vi "fft_test.vi"() -> ()   [LabVIEW 2016]
uses:
  xcontrol/Start Button.xctl
  <vilib>/silver_ctls/ArrayMatrixCluster/Real Matrix NI_Silver.ctl
  <vilib>/Instr/_visa.llb/VISA Configure Serial Port (Instr).vi
  <instrlib>/Tektronix TDS 200 1000 2000 Series/Public/Data/Read (Single Waveform).vi
  <instrlib>/Tektronix TDS 200 1000 2000 Series/Tektronix TDS 200 1000 2000 Series.lvlib
panel:
  out "OSC ERR":bool=TRUE
  in  "Vertical Range (10.0 V/div)":dbl=0.005 format="%^1_3g"
  out "Waveform Graph":dbl[](graph)
  in  "Sampling Frequency":dbl=500000.0
  in  "Number of Sample":i32=2500
  out "Ölçülen Sinyal":dynamicdata(graph)
  out "Real Matrix":T1
  out "İlk Ayar":bool=TRUE
  out "Osc Data":waveform(dbl)(graph)
  in  "Osiloskop Portu":refnum<visa-resource-name>="USB0::0x0699::0x0363::C102985::INSTR"
  in  "Start Button":dbl(xcontrol)
  in  "Frekans (kHz)":i32(slide)=100 caption="Amplitude(V)" step=1 scale=0.0..100.0
  in  "Reset Dafault":bool
  in  "Teta":i32(slide) scale=0.0..360.0
  in  "Sinyal Jeneratörü Portu":refnum<visa-resource-name>="COM4"
  in  "OUTPUT":bool=TRUE caption="Output"
  in  "Offset":i32(slide) scale=0.0..10.0
  in  "Amplitude(V)":i32(slide)=20 scale=0.0..20.0
  in  "cmdOrjin":bool
  in  "cmdStop":bool
  # "R-O Tarayıcı ile Bilgisayar Kontrollü Halka Anten Radyasyon Paterni Ölçüm Düzeneği Geliştirilmesi"
  # "Frekans"
  # "Teta"
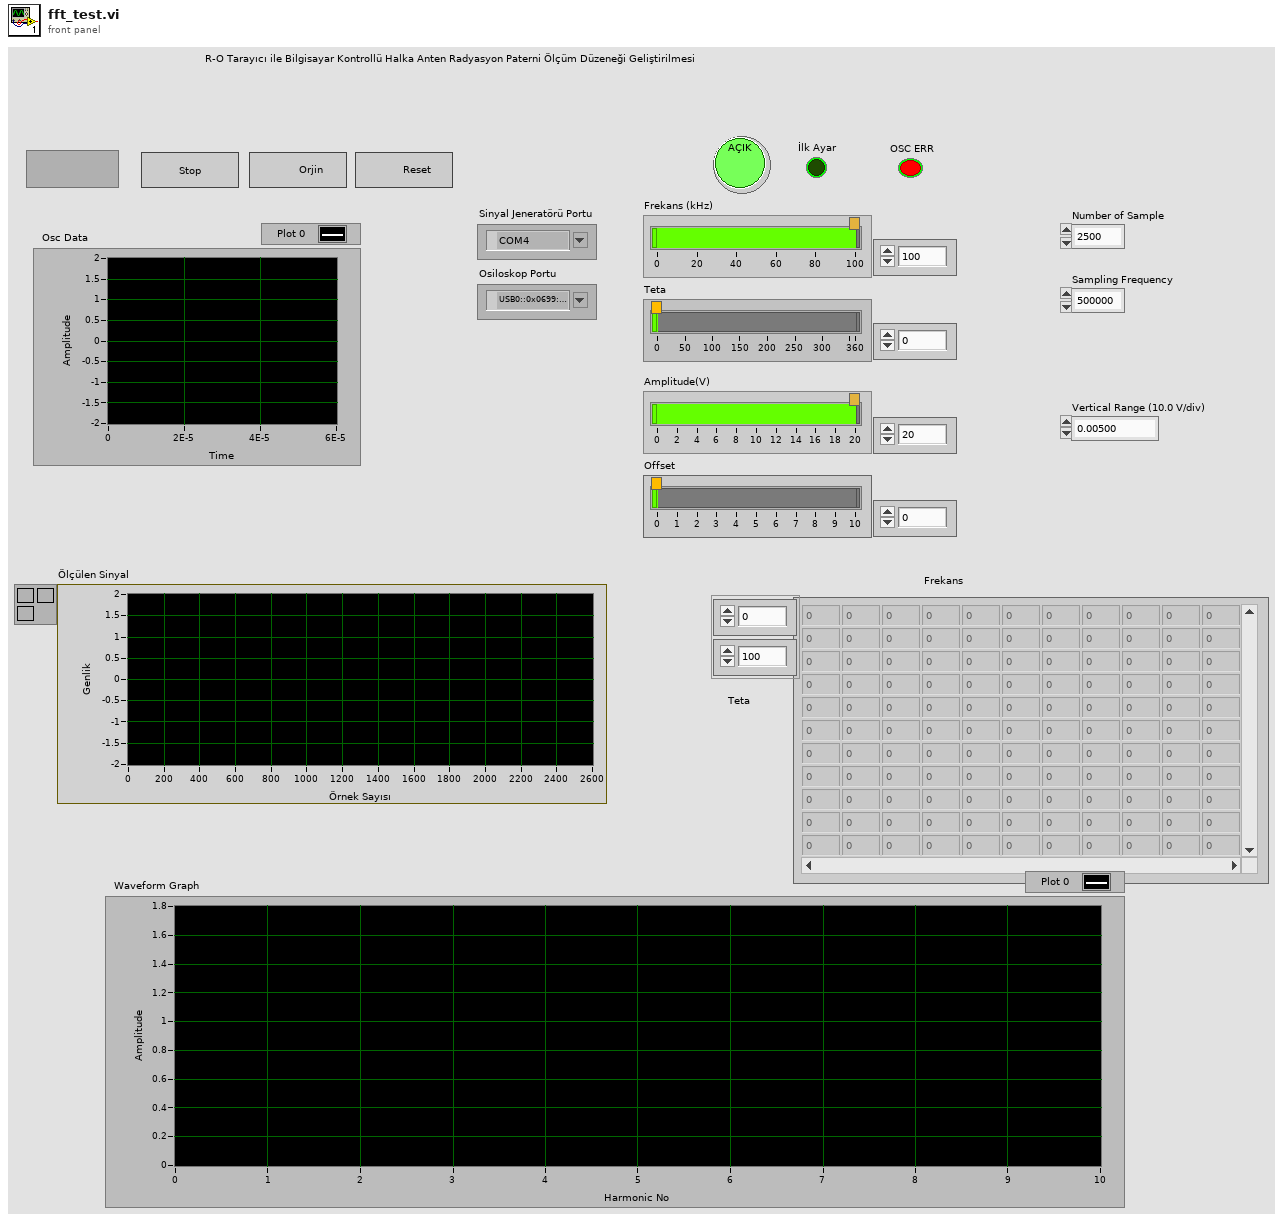
[diagram p1: front panel]
types:
  T1 = typedef "Real Matrix NI_Silver.ctl" = dbl[][]
  T2 = cluster{"Baud Rate":u32, "Parity":u16, "Stop Bits":u16, "Flow Control":u16}
  T3 = typedef "NI_Matrix.lvlib/RealMatrix.ctl" = dbl[][]
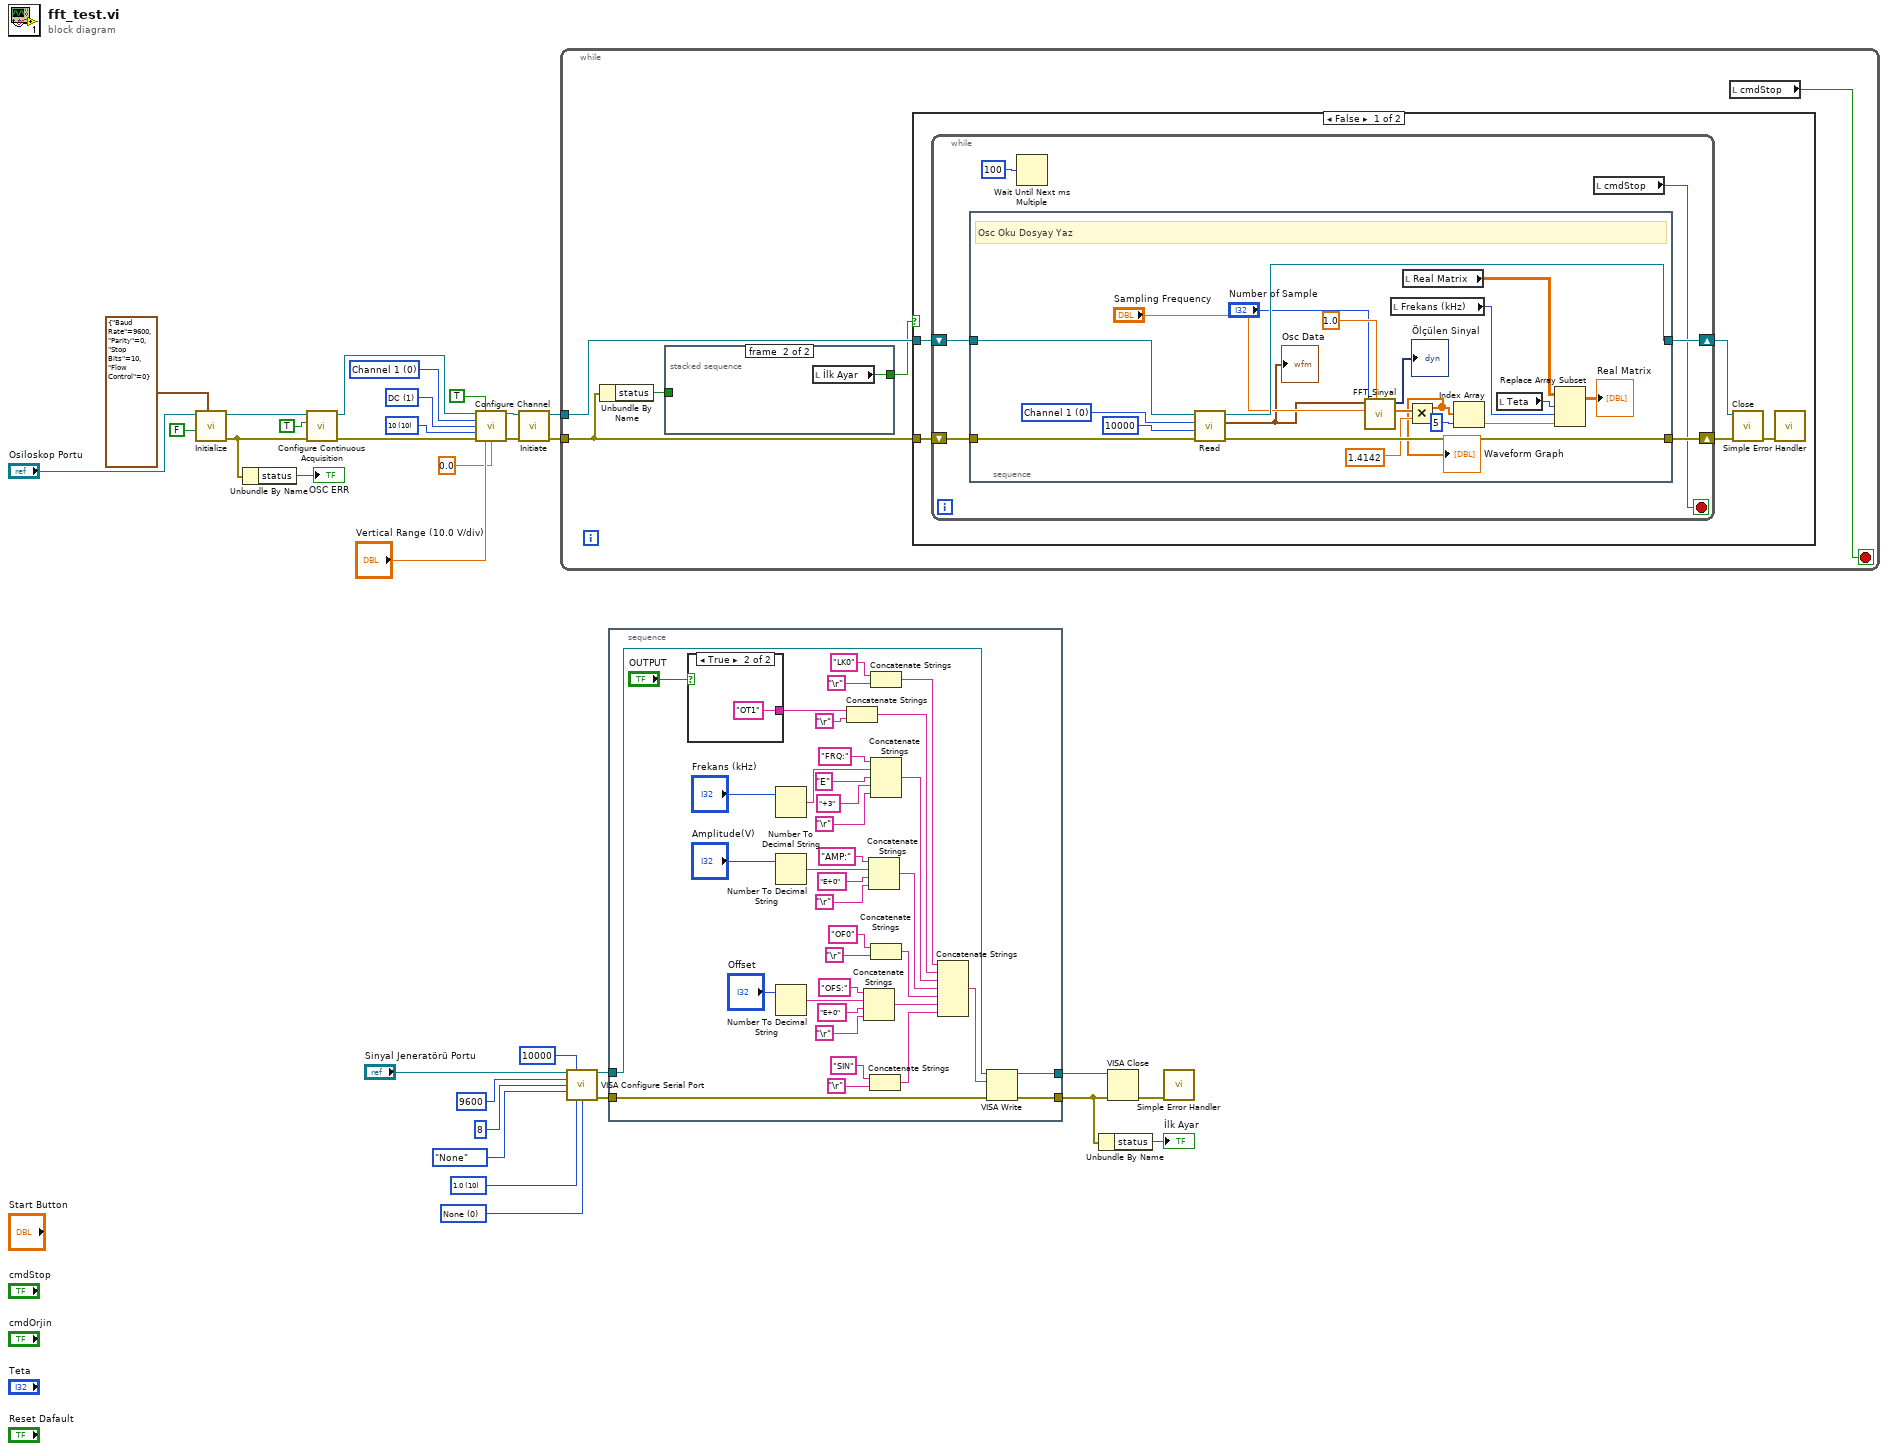
[diagram p0: block diagram]
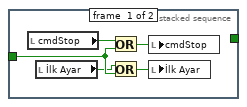
[diagram p2: hidden frame]
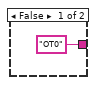
[diagram p4: hidden frame]
diagram:
  w13 = 1 items=["AC", "DC", "Ground"] ("Vertical Coupling (1: DC)")
  w14 = 0 items=["Channel 1", "Channel 2", "Channel 3", "Channel 4", "Math", "Reference A", "Reference B", "Reference C", "Reference D"] ("Channel (0: Channel 1)")
  w16 = 10 items=["1"=1, "10"=10, "20"=20, "50"=50, "100"=100, "500"=500, "1000"=1000] ("Probe Attenuation (10: 10X)")
  w32 = u16 0 items=["None", "XON/XOFF", "RTS/CTS", "XON/XOFF & RTS/CTS", "DTR/DSR", "XON/XOFF & DTR/DSR"] ("flow control (0:none)")
  w31 = u16 10 items=["1.0"=10, "1.5"=15, "2.0"=20] ("stop bits (10: 1 bit)")
  n1 = call <instrlib>:"Initialize.vi"("Serial Configuration"=T2 {"Baud Rate"=9600, "Parity"=0, "Stop Bits"=10, "Flow Control"=0} ("Osiloskop Config"), "Reset? (T: Yes)"=FALSE, "VISA resource name"="Osiloskop Portu") -> ("error out"=w2:errorcluster, "VISA resource name out"=w5:refnum<visa-resource-name>)  [unwired: 2 in, 5 out]
  n2 = Unbundle By Name(w2) -> ("status"=→"OSC ERR":bool)
  n3 = call <instrlib>:"Configure Continuous Acquisition.vi"("error in (no error)"=w2, "Enable Continuous Acquisition Mode (True)"=TRUE, "VISA resource name"=w5) -> ("error out"=w17:errorcluster, "VISA resource name out"=w20:refnum<visa-resource-name>)  [unwired: 7 out]
  n4 = call <instrlib>:"Configure Channel.vi"("VISA resource name"=w20, "Enable Channel (True)"=TRUE, "Channel (0: Channel 1)"=w14, "Vertical Coupling (1: DC)"=w13, "Probe Attenuation (10: 10X)"=w16, "error in (no error)"=w17, "Vertical Range (10.0 V/div)"="Vertical Range (10.0 V/div)", "Vertical Offset (0.0 divs)"=0.0) -> ("VISA resource name out"=w19:refnum<visa-resource-name>, "error out"=w18:errorcluster)  [unwired: 6 in]
  n5 = call <instrlib>:"Initiate.vi"("error in (no error)"=w18, "VISA resource name"=w19) -> ("error out"=w21:errorcluster, "VISA resource name out"=w22:refnum<visa-resource-name>)  [unwired: 8 out]
  n6 = while {
    tunnel: w22 -> [w37]
    tunnel: w21 -> [w36]
    stop <- w33 stop-if-true
    n7 = Unbundle By Name(w36) -> ("status"=w35:bool)
    n8 = stacked-sequence {
      tunnel: w35 -> [w39 _]
      tunnel: [_ w43] -> w34
      frame #0 {
        n9 = local read "cmdStop"() -> (w41:bool)
        n10 = local read "İlk Ayar"() -> (w38:bool)
        n11 = Or(x=w41, y=w39) -> (x .or. y?=w42:bool)
        n12 = Or(x=w38, y=w39) -> (x .or. y?=w40:bool)
        n13 = local write "cmdStop"(w42) -> ()
        n14 = local write "İlk Ayar"(w40) -> ()
      }
      frame #1 {
        n15 = local read "İlk Ayar"() -> (w43:bool)
      }
    }
    n16 = case shown="False" w34 {
      tunnel: w37 -> [w48 _]
      tunnel: w36 -> [w47 _]
      frame False {
        n17 = while {
          shift-right: [w52] -> w46
          shift-left: w48 -> [w54]
          shift-right: [w51] -> w45
          shift-left: w47 -> [w53]
          stop <- w49 stop-if-true
          n18 = stacked-sequence {
            tunnel: w54 -> [w64]
            tunnel: w53 -> [w63]
            tunnel: [w72] -> w51
            tunnel: [w71] -> w52
            frame #0 {
              w73 = u16 0 items=["Channel 1", "Channel 2", "Channel 3", "Channel 4", "Math", "Reference A", "Reference B", "Reference C", "Reference D"] ("Channel B (1: Channel 2)")
              # "Osc Oku Dosyay Yaz"
              n19 = call-poly <instrlib>:"Read.vi"("error in (no error)"=w63, "Timeout (10000 ms)"=u32 10000 ("Timeout (10000 ms) 2"), "Source (0: Channel 1)"=w73, "VISA resource name"=w64) -> ("error out"=w72:errorcluster, "Waveform Data"=w59:waveform(dbl), "VISA resource name out"=w71:refnum<visa-resource-name>)  [unwired: 5 out]
              "Osc Data" <- w59
              n20 = call "FFT_Sinyal.vi"("Oran"=1.0, "Number of Sample"="Number of Sample", "Sampling Frequency"="Sampling Frequency", "Sinyal"=w59) -> ("Sinyal Genlik"=w57:dbl[], "Ölçülen Sinyal"=→"Ölçülen Sinyal":dynamicdata)  [unwired: 2 in, 2 out]
              n21 = local read "Frekans (kHz)"() -> (w66:i32)
              n22 = local read "Real Matrix"() -> (w69:T1)
              n23 = Multiply(x=w57, y=1.4142) -> (x*y=w55:dbl[])
              "Waveform Graph" <- w55
              n24 = Index Array(array=w55, index=5) -> (element=w67:dbl)
              n25 = local read "Teta"() -> (w65:i32)
              n26 = Replace Array Subset ("Set Matrix Elements")(array=w69, new element=w67, index (row)=w65, index (col)=w66) -> (→"Real Matrix":T3)
            }
          }
          n27 = Wait Until Next ms Multiple(millisecond multiple=u32 100) -> ()  [unwired: 1 out]
          n28 = local read "cmdStop"() -> (w49:bool)
        }
        n29 = call <instrlib>:"Close.vi"("error in (no error)"=w45, "VISA resource name"=w46) -> ("error out"=w44:errorcluster)  [unwired: 9 in]
        n30 = call <vilib>:"Simple Error Handler.vi"("error in (no error)"=w44) -> ()  [unwired: 4 in, 5 out]
      }
      frame True {
      }
    }
    n31 = local read "cmdStop"() -> (w33:bool)
  }
  n32 = call-poly "VISA Configure Serial Port"("VISA resource name"="Sinyal Jeneratörü Portu", "timeout (10sec)"=u32 10000, "baud rate (9600)"=u32 9600, "data bits (8)"=u16 8, "parity (0:none)"=enum16{"None", "Odd", "Even", "Mark", "Space"}."None", "stop bits (10: 1 bit)"=w31, "flow control (0:none)"=w32) -> ("VISA resource name out"=w11:refnum<visa-resource-name>, "error out"=w10:errorcluster)  [unwired: 7 in]
  n33 = stacked-sequence {
    tunnel: w11 -> [w78]
    tunnel: w10 -> [w77]
    tunnel: [w76] -> w9
    tunnel: [w75] -> w6
    frame #0 {
      n34 = case shown="True" "OUTPUT" {
        tunnel: ["OT0" "OT1"] -> w105
        frame False {
        }
        frame True {
        }
      }
      n35 = Number To Decimal String(number="Frekans (kHz)") -> (decimal integer string=w100:string)  [unwired: 1 in]
      n36 = Number To Decimal String(number="Amplitude(V)") -> (decimal integer string=w94:string)  [unwired: 1 in]
      n37 = Number To Decimal String(number="Offset") -> (decimal integer string=w87:string)  [unwired: 1 in]
      n38 = Concatenate Strings(w105, "\r") -> (w102:string)
      n39 = Concatenate Strings("OFS:", w87, "E+0", "\r") -> (w86:string)
      n40 = Concatenate Strings("AMP:", w94, "E+0", "\r") -> (w93:string)
      n41 = Concatenate Strings("SIN", "\r") -> (w85:string)
      n42 = Concatenate Strings("LK0", "\r") -> (w103:string)
      n43 = Concatenate Strings("FRQ:", w100, "E", "+3", "\r") -> (w99:string)
      n44 = Concatenate Strings("OF0", "\r") -> (w90:string)
      n45 = Concatenate Strings(w103, w102, w99, w93, w90, w86, w85) -> (w79:string)
      n46 = VISA Write(VISA resource name=w78, write buffer=w79, error in (no error)=w77) -> (VISA resource name out=w76:refnum<visa-resource-name>, error out=w75:errorcluster)  [unwired: 1 out]
    }
  }
  n47 = Unbundle By Name(w6) -> ("status"=→"İlk Ayar":bool)
  n48 = VISA Close(VISA resource name=w9, error in (no error)=w6) -> (error out=w8:errorcluster)
  n49 = call <vilib>:"Simple Error Handler.vi"("error in (no error)"=w8) -> ()  [unwired: 4 in, 5 out]
